vi "read_P_Dop_relays.vi"() -> (0 "P_Dop Gas Source":bool, 1 "P_Dop H2 Dilute":bool, 2 "P_Dop Remote":bool, 3 "P_Dop Run":bool, 4 "P_Dop Bubbler":bool, 5 "P_Dop Active":bool)   [LabVIEW 2011]
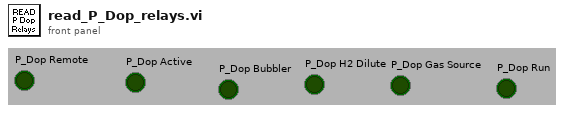
[diagram p1: front panel]
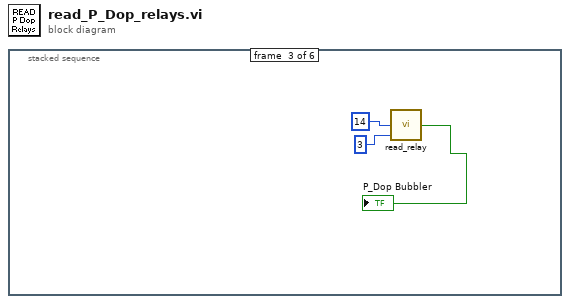
[diagram p0: block diagram]
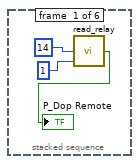
[diagram p2: hidden frame]
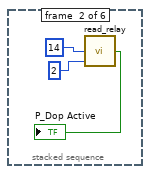
[diagram p3: hidden frame]
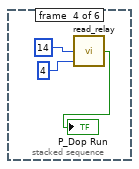
[diagram p4: hidden frame]
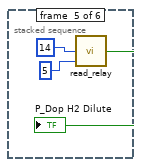
[diagram p5: hidden frame]
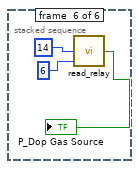
[diagram p6: hidden frame]
diagram:
  n1 = stacked-sequence {
    frame #0 {
      n2 = call "read_relay.vi"("Relay"=1, "Slot"=14) -> ("Relay Status"=→"P_Dop Remote":bool)  [unwired: 1 out]
    }
    frame #1 {
      n3 = call "read_relay.vi"("Relay"=2, "Slot"=14) -> ("Relay Status"=→"P_Dop Active":bool)  [unwired: 1 out]
    }
    frame #2 {
      n4 = call "read_relay.vi"("Relay"=3, "Slot"=14) -> ("Relay Status"=→"P_Dop Bubbler":bool)  [unwired: 1 out]
    }
    frame #3 {
      n5 = call "read_relay.vi"("Relay"=4, "Slot"=14) -> ("Relay Status"=→"P_Dop Run":bool)  [unwired: 1 out]
    }
    frame #4 {
      n6 = call "read_relay.vi"("Relay"=5, "Slot"=14) -> ("Relay Status"=→"P_Dop H2 Dilute":bool)  [unwired: 1 out]
    }
    frame #5 {
      n7 = call "read_relay.vi"("Relay"=6, "Slot"=14) -> ("Relay Status"=→"P_Dop Gas Source":bool)  [unwired: 1 out]
    }
  }
